vi "MainUI.vi"() -> ()   [LabVIEW 2016]
uses:
  Package Libraries/Message Queue/private/MessageQueue.MessageTypeDef.ctl
  Package ErrorHandling/ErrorHandling.lvclass/ErrorHandling.ctl
  Package ResourceControl/ViHandler/ViHandler.RunModes.ctl
  Package ErrorHandling/ErrorHandling.checkForErrorAndHandle.vi
  Package ErrorHandling/ErrorHandling.GetErrorHandler.vi
  <vilib>/Utility/error.llb/Clear Errors.vi
  Package Libraries/StringFunctions/StringFunctions_ReplaceAllBlindSigns.vi
  <vilib>/dlg_ctls.llb/Space Constant.vi
  Package Libraries/TimingFunctions/TimingFunctions_getUtcTimestamp.vi
  <vilib>/Utility/error.llb/Trim Whitespace.vi
  <vilib>/Utility/error.llb/Search and Replace Pattern.vi
  Package ErrorHandling/ErrorHandling.addLastErrorToFile.vi
  Package Simulation/Simulation Main/Simulation.Main.vi
  <vilib>/Utility/error.llb/Error Cluster From Error Code.vi
  Package ErrorHandling/ErrorHandling.lvclass
  <vilib>/ErrorRing/Error Ring.xnode
  Package ResourceControl/ViHandler/ViHandler.lvclass
  Package ResourceControl/ObjectHandler/ObjectHandler.lvclass
  Package Simulation/Simulation Main/Simulation.lvclass
panel:
  out "LastLoaded":string="LoadImportAssistant"
  out "NowLoaded":string="LoadImportAssistant"
  in  "PlaceHolder2Btn":bool
  in  "ParameterBtn":bool
  in  "ManualBtn":bool
  in  "DebugBtn":bool
  in  "ErrorHistoryBtn":bool
  in  "SimulationBtn":bool
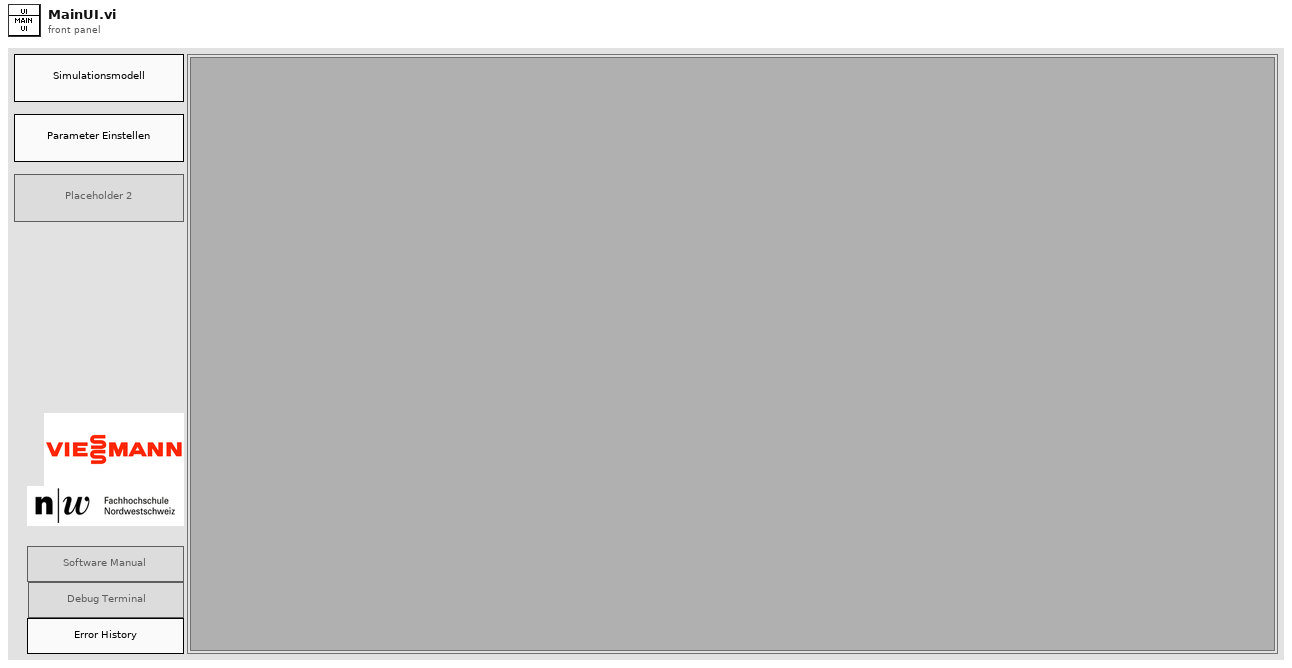
[diagram p1: front panel]
types:
  T1 = typedef "MessageQueue.MessageTypeDef.ctl" = cluster{"Message":string, "Data":variant}
  T2 = enum32{"Invalid", "Standard", "Closed", "Hidden", "Minimized", "Maximized"}
  T3 = enum8{"Enabled", "Disabled", "Disabled and Grayed Out"}
  T4 = typedef "ViHandler.lvclass/ViHandler.RunModes.ctl" = enum16{"FP Closed", "FP Open", "FP Open, Centered"}
  T5 = typedef "ViHandler.lvclass/ViHandler.ViInfo.ctl" = cluster{"ViName":string, "ViReference":refnum<vi>, "ViQueueName":string}
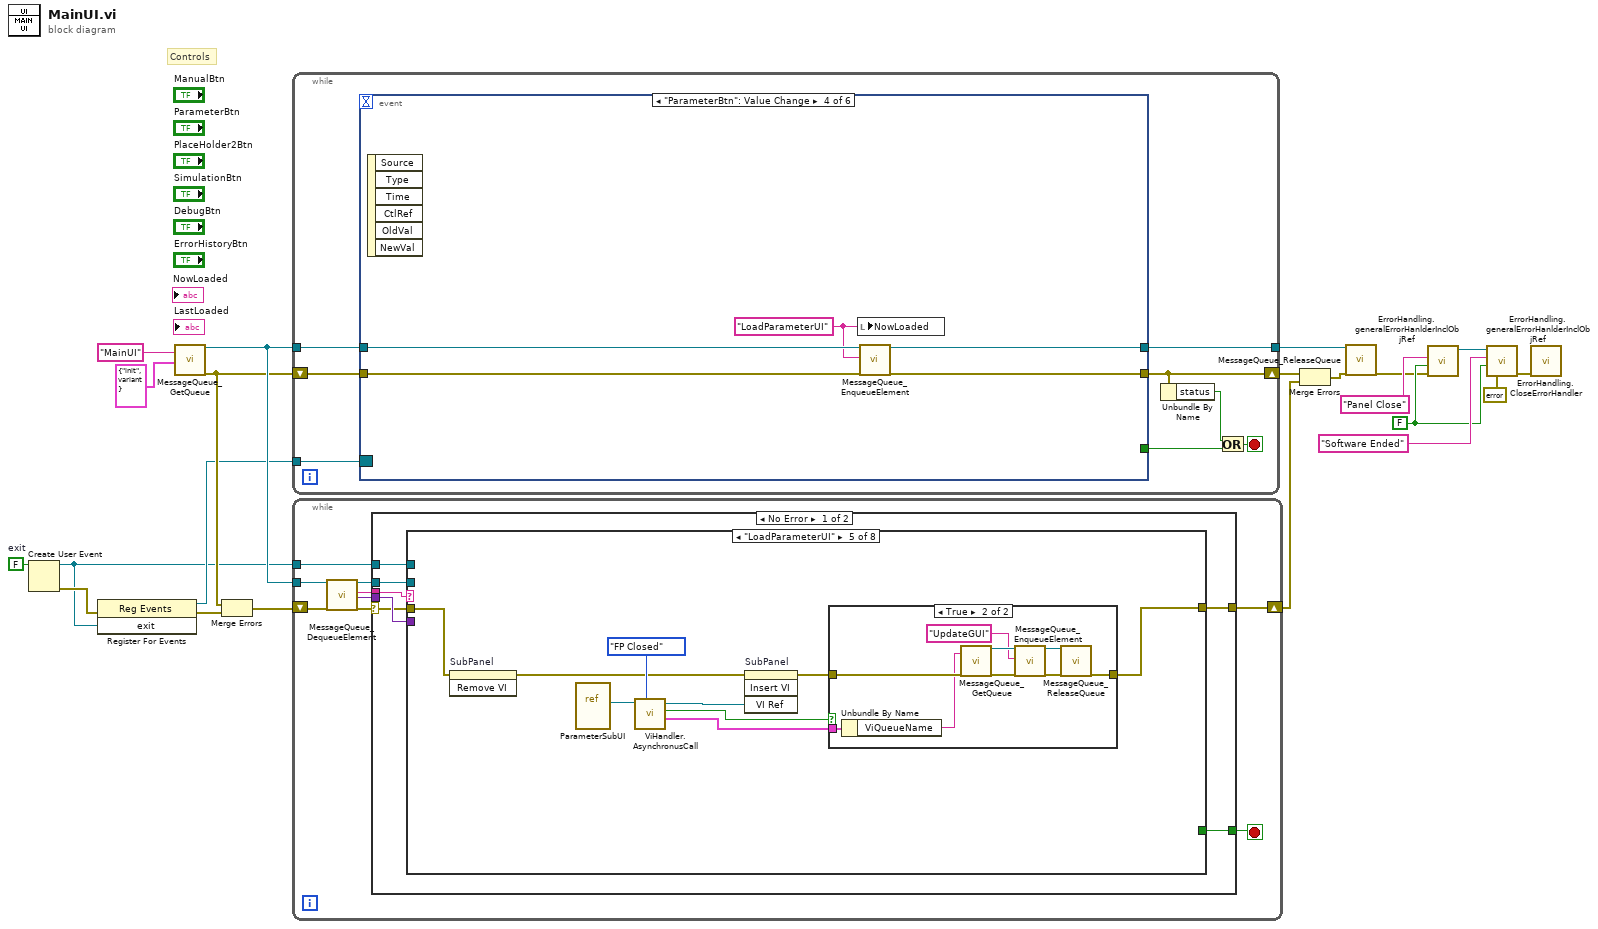
[diagram p0: block diagram]
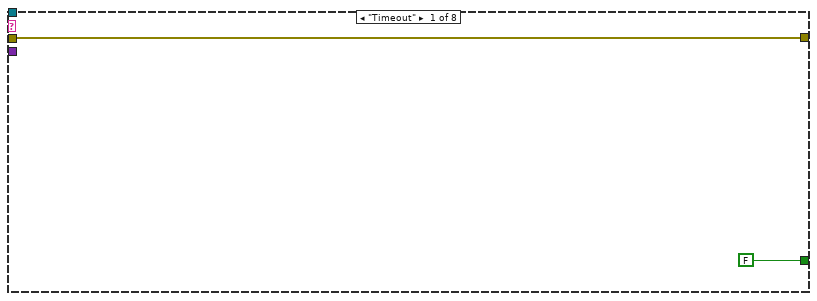
[diagram p2: hidden frame]
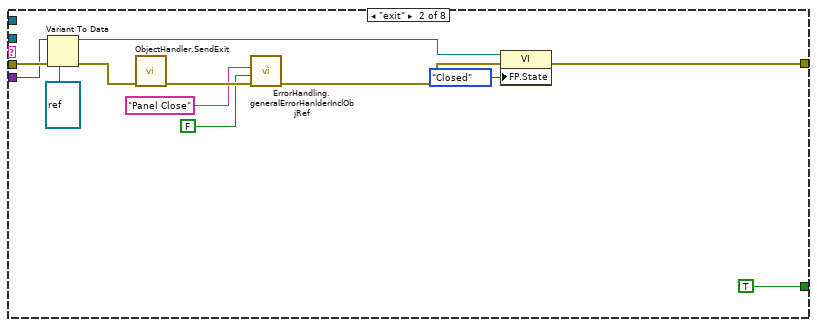
[diagram p3: hidden frame]
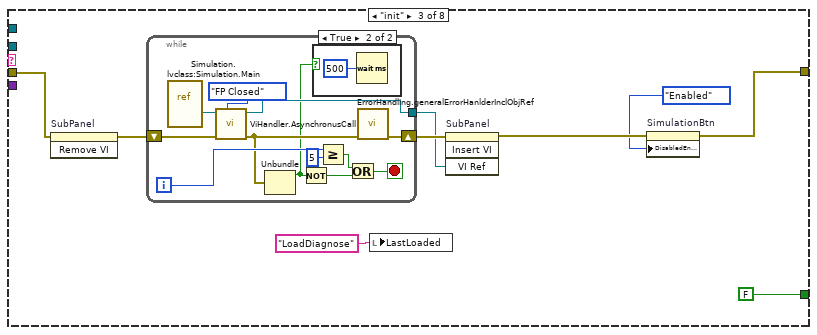
[diagram p4: hidden frame]
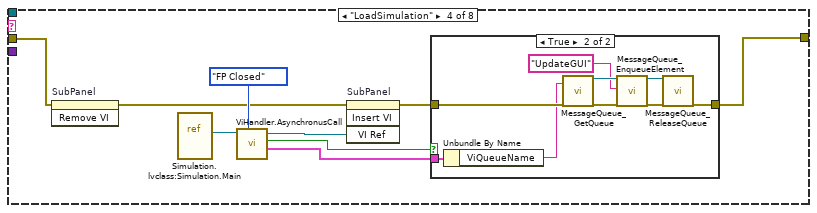
[diagram p6: hidden frame]
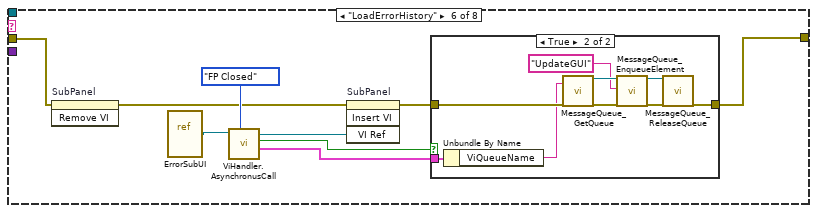
[diagram p9: hidden frame]
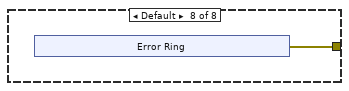
[diagram p12: hidden frame]
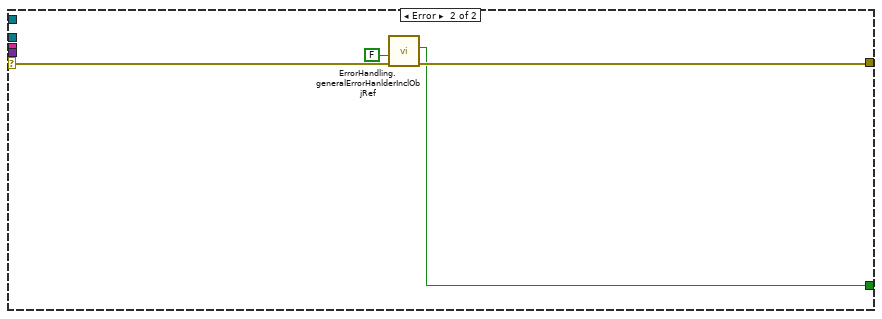
[diagram p13: hidden frame]
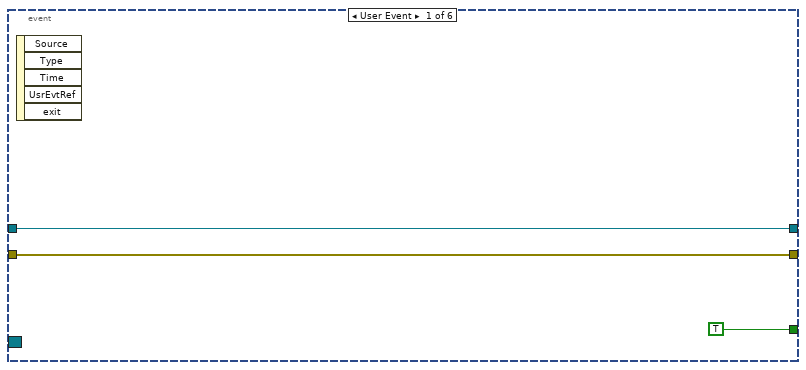
[diagram p14: hidden frame]
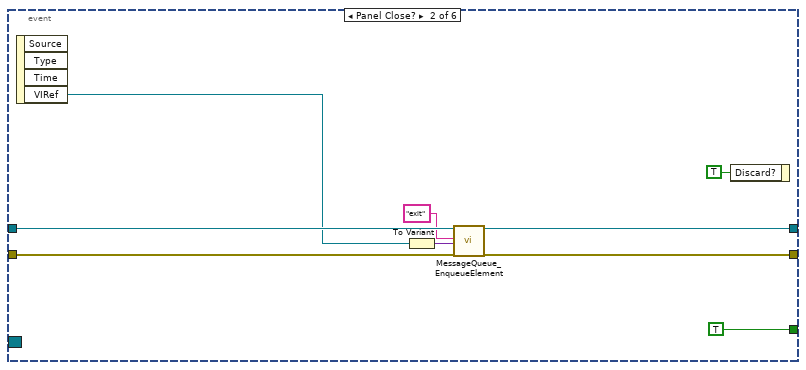
[diagram p15: hidden frame]
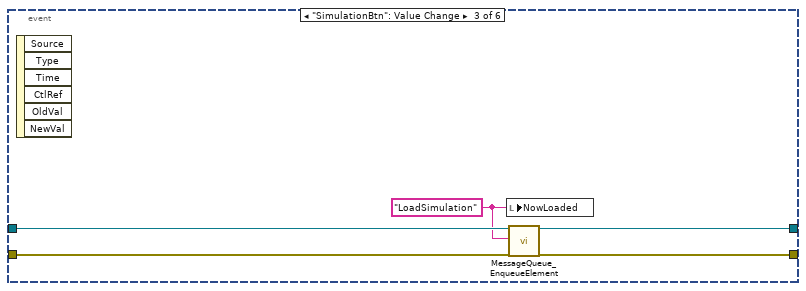
[diagram p16: hidden frame]
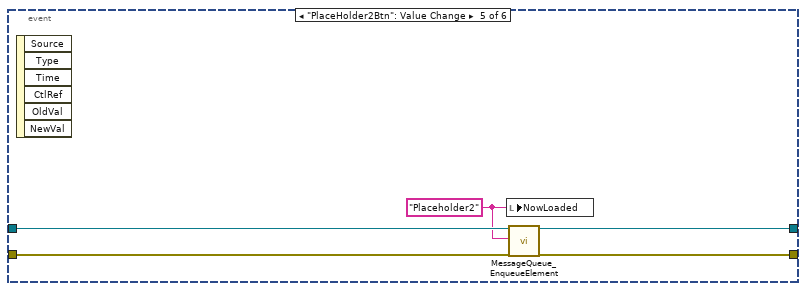
[diagram p17: hidden frame]
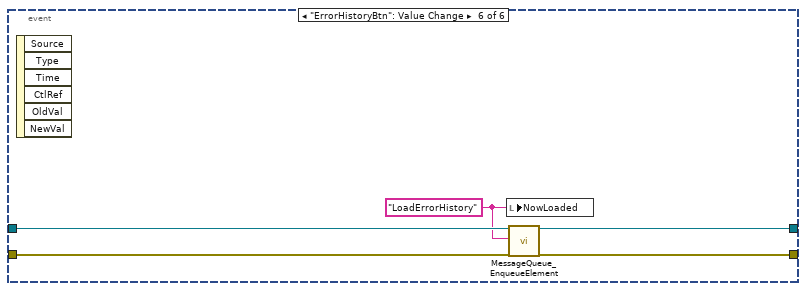
[diagram p18: hidden frame]
diagram:
  w3 = FALSE ("StopOnError")
  w14 = FALSE  # exit
  # "Controls"
  n1 = Create User Event(user event datatype=w14) -> (user event=w12:refnum<user-event>, error out=w13:errorcluster)  [unwired: 1 in]
  n2 = register-events(error in=w13, w12) -> (reference out=w16:refnum<event-registration>, error out=w18:errorcluster)  [unwired: 1 in]
  n3 = call "MessageQueue_GetQueue.vi"("Name"="MainUI", "OptionalInitValue"=T1 {"Message"="init", "Data"=variant}) -> ("QueueOut"=w20:refnum<queue>, "ErrorOut"=w17:errorcluster)  [unwired: 15 in, 1 out]
  n4 = Merge Errors(w17, w18) -> (w15:errorcluster)
  n5 = while {
    tunnel: w20 -> [w29]
    tunnel: [w28] -> w21
    shift-right: [w25] -> w9
    shift-left: w17 -> [w27]
    tunnel: w16 -> [w22]
    stop <- w24 stop-if-true
    n6 = event shown="[3] \"ParameterBtn\": Value Change" {
      selector: w22 -> [_ _ _ _ _ _]
      dyn-events: _ -> [_ _ _ _ _ _]
      timeout: _ -> [_ _ _ _ _ _]
      tunnel: w29 -> [w31 w41 w44 w49 w54 w59]
      tunnel: [w31 w40 w46 w51 w56 w61] -> w28
      tunnel: [w30 w33 w45 w50 w55 w60] -> w25
      tunnel: w27 -> [w30 w36 w43 w48 w53 w58]
      tunnel: [TRUE TRUE _ _ _ _] -> w26
      event User Event {
        n7 = event-data() -> ()  [unwired: 1 in, 5 out]
      }
      event Panel Close? {
        n8 = event-data() -> ("VIRef"=w34:refnum<vi>)  [unwired: 1 in, 3 out]
        n9 = To Variant(anything=w34) -> (Variant=w35:variant)
        n10 = call "MessageQueue_EnqueueElement.vi"("QueueIn"=w41, "Message"="exit", "Data"=w35, "ErrorIn"=w36) -> ("QueueOut"=w40:refnum<queue>, "ErrorOut"=w33:errorcluster)  [unwired: 14 in]
        n11 = event-data("Discard?"=TRUE) -> ()  [unwired: 1 in, 1 out]
      }
      event "SimulationBtn": Value Change {
        w42 = "LoadSimulation" ("Message")
        n12 = event-data() -> ()  [unwired: 1 in, 6 out]
        n13 = local write "NowLoaded"(w42) -> ()
        n14 = call "MessageQueue_EnqueueElement.vi"("QueueIn"=w44, "Message"=w42, "ErrorIn"=w43) -> ("QueueOut"=w46:refnum<queue>, "ErrorOut"=w45:errorcluster)  [unwired: 15 in]
      }
      event "ParameterBtn": Value Change {
        w47 = "LoadParameterUI" ("Message")
        n15 = event-data() -> ()  [unwired: 1 in, 6 out]
        n16 = local write "NowLoaded"(w47) -> ()
        n17 = call "MessageQueue_EnqueueElement.vi"("QueueIn"=w49, "Message"=w47, "ErrorIn"=w48) -> ("QueueOut"=w51:refnum<queue>, "ErrorOut"=w50:errorcluster)  [unwired: 15 in]
      }
      event "PlaceHolder2Btn": Value Change {
        w52 = "Placeholder2" ("Message")
        n18 = event-data() -> ()  [unwired: 1 in, 6 out]
        n19 = local write "NowLoaded"(w52) -> ()
        n20 = call "MessageQueue_EnqueueElement.vi"("QueueIn"=w54, "Message"=w52, "ErrorIn"=w53) -> ("QueueOut"=w56:refnum<queue>, "ErrorOut"=w55:errorcluster)  [unwired: 15 in]
      }
      event "ErrorHistoryBtn": Value Change {
        w57 = "LoadErrorHistory" ("Message")
        n21 = event-data() -> ()  [unwired: 1 in, 6 out]
        n22 = local write "NowLoaded"(w57) -> ()
        n23 = call "MessageQueue_EnqueueElement.vi"("QueueIn"=w59, "Message"=w57, "ErrorIn"=w58) -> ("QueueOut"=w61:refnum<queue>, "ErrorOut"=w60:errorcluster)  [unwired: 15 in]
      }
    }
    n24 = Unbundle By Name(w25) -> ("status"=w23:bool)
    n25 = Or(x=w23, y=w26) -> (x .or. y?=w24:bool)
  }
  n26 = while {
    tunnel: w20 -> [w70]
    tunnel: w12 -> [w63]
    shift-right: [w62] -> w10
    shift-left: w15 -> [w64]
    stop <- w65 stop-if-true
    n27 = call "MessageQueue_DequeueElement.vi"("QueueIn"=w70, "ErrorIn"=w64) -> ("QueueOut"=w68:refnum<queue>, "Message"=w67:string, "Data"=w66:variant, "ErrorOut"=w69:errorcluster)  [unwired: 13 in, 1 out]
    n28 = case shown="No Error" w69 {
      selector: w69 -> [w73 w181]
      tunnel: w68 -> [w77 _]
      tunnel: w67 -> [w76 _]
      tunnel: w66 -> [w75 _]
      tunnel: [w74 w179] -> w65
      tunnel: w63 -> [w72 _]
      tunnel: [w71 w180] -> w62
      frame No Error {
        n29 = case shown="\"LoadParameterUI\"" w76 {
          tunnel: w77 -> [_ _ _ _ _ _ _ _]
          tunnel: w75 -> [_ w83 _ _ _ _ _ _]
          tunnel: [FALSE TRUE FALSE _ _ _ _ _] -> w74
          tunnel: w73 -> [w78 w85 w94 w117 w136 w155 w171 _]
          tunnel: w72 -> [_ _ _ _ _ _ _ _]
          tunnel: [w78 w80 w93 w116 w135 w154 w171 w172] -> w71
          frame "Timeout" {
          }
          frame "exit" {
            n30 = Variant To Data(error in=w85, type=refnum<vi> refnum ("VIRef"), Variant=w83) -> (data=w81:refnum<vi>, error out=w84:errorcluster)
            n31 = call "ObjectHandler.SendExit.vi"("ErrorIn"=w84) -> ("ErrorOut"=w89:errorcluster)  [unwired: 10 in]
            n32 = call "ErrorHandling.generalErrorHanlderInclObjRef.vi"("error in"=w89, "StopOnError"=FALSE, "Comment(optional)"="Panel Close" ("Comment")) -> ("error out"=w88:errorcluster)  [unwired: 6 in, 2 out]
            n33 = property class="VI"(reference=w81, error in=w88, "FP.State"=T2."Closed" ("Front Panel Window:State")) -> (error out=w80:errorcluster)  [unwired: 1 out]
          }
          frame "init" {
            n34 = invoke on="SubPanel" class="SubPnl" method="Remove VI"(error in=w94) -> (error out=w96:errorcluster)  [unwired: 2 in, 2 out]
            n35 = while {
              tunnel: [w102] -> w95
              shift-right: [w103] -> w97
              shift-left: w96 -> [w110]
              i -> [w107]
              stop <- w105 stop-if-true
              n36 = vi-ref "Simulation.lvclass:Simulation.Main.vi"() -> (w112:refnum<vi>)
              n37 = call "ViHandler.AsynchronusCall.vi"("Modes"=ViHandler.RunModes."FP Closed", "Error In"=w110, "ViReference"=w112) -> ("error out"=w104:errorcluster, "ViReference"=w102:refnum<vi>)  [unwired: 5 in, 2 out]
              n38 = Unbundle(w104) -> ("status"=w101:bool)  [unwired: 2 out]
              n39 = Not(x=w101) -> (.not. x?=w109:bool)
              n40 = case shown="True" w101 {
                frame False {
                }
                frame True {
                  n41 = Wait (ms)(milliseconds to wait=u32 500) -> ()  [unwired: 1 out]
                }
              }
              n42 = Greater Or Equal?(x=w107, y=5) -> (x >= y?=w108:bool)
              n43 = Or(x=w108, y=w109) -> (x .or. y?=w105:bool)
              n44 = call "ErrorHandling.generalErrorHanlderInclObjRef.vi"("error in"=w104) -> ("error out"=w103:errorcluster)  [unwired: 8 in, 2 out]
            }
            n45 = local write "LastLoaded"("LoadDiagnose" ("Message")) -> ()
            n46 = invoke on="SubPanel" class="SubPnl" method="Insert VI"(error in=w97, "VI Ref"=w95) -> (error out=w99:errorcluster)  [unwired: 2 in, 3 out]
            n47 = property on="SimulationBtn" class="Bool"(error in=w99, "DisabledEnum"=T3."Enabled" ("Disabled")) -> (error out=w93:errorcluster)  [unwired: 1 in, 1 out]
          }
          frame "LoadSimulation" {
            n48 = invoke on="SubPanel" class="SubPnl" method="Remove VI"(error in=w117) -> (error out=w118:errorcluster)  [unwired: 2 in, 2 out]
            n49 = vi-ref "Simulation.lvclass:Simulation.Main.vi"() -> (w115:refnum<vi>)
            n50 = call "ViHandler.AsynchronusCall.vi"("Modes"=ViHandler.RunModes."FP Closed", "ViReference"=w115) -> ("ViInfo(OnlyIfFound=true)"=w122:T5, "ViFound?"=w121:bool, "ViReference"=w114:refnum<vi>)  [unwired: 6 in, 1 out]
            n51 = invoke on="SubPanel" class="SubPnl" method="Insert VI"(error in=w118, "VI Ref"=w114) -> (error out=w120:errorcluster)  [unwired: 2 in, 3 out]
            n52 = case shown="True" w121 {
              tunnel: w120 -> [w123 w132]
              tunnel: [w123 w129] -> w116
              tunnel: w122 -> [_ w128]
              frame False {
              }
              frame True {
                n53 = Unbundle By Name(w128) -> ("ViQueueName"=w125:string)
                n54 = call "MessageQueue_GetQueue.vi"("Name"=w125, "ErrorIn"=w132) -> ("QueueOut"=w127:refnum<queue>, "ErrorOut"=w131:errorcluster)  [unwired: 15 in, 1 out]
                n55 = call "MessageQueue_EnqueueElement.vi"("QueueIn"=w127, "Message"="UpdateGUI", "ErrorIn"=w131) -> ("QueueOut"=w126:refnum<queue>, "ErrorOut"=w130:errorcluster)  [unwired: 15 in]
                n56 = call "MessageQueue_ReleaseQueue.vi"("QueueIn"=w126, "ErrorIn"=w130) -> ("ErrorOut"=w129:errorcluster)  [unwired: 15 in, 2 out]
              }
            }
          }
          frame "LoadParameterUI" {
            n57 = invoke on="SubPanel" class="SubPnl" method="Remove VI"(error in=w136) -> (error out=w137:errorcluster)  [unwired: 2 in, 2 out]
            n58 = vi-ref "ParameterSubUI.vi"() -> (w134:refnum<vi>)
            n59 = call "ViHandler.AsynchronusCall.vi"("Modes"=ViHandler.RunModes."FP Closed", "ViReference"=w134) -> ("ViInfo(OnlyIfFound=true)"=w141:T5, "ViFound?"=w140:bool, "ViReference"=w133:refnum<vi>)  [unwired: 6 in, 1 out]
            n60 = invoke on="SubPanel" class="SubPnl" method="Insert VI"(error in=w137, "VI Ref"=w133) -> (error out=w139:errorcluster)  [unwired: 2 in, 3 out]
            n61 = case shown="True" w140 {
              tunnel: w139 -> [w142 w151]
              tunnel: [w142 w148] -> w135
              tunnel: w141 -> [_ w147]
              frame False {
              }
              frame True {
                n62 = Unbundle By Name(w147) -> ("ViQueueName"=w144:string)
                n63 = call "MessageQueue_GetQueue.vi"("Name"=w144, "ErrorIn"=w151) -> ("QueueOut"=w146:refnum<queue>, "ErrorOut"=w150:errorcluster)  [unwired: 15 in, 1 out]
                n64 = call "MessageQueue_EnqueueElement.vi"("QueueIn"=w146, "Message"="UpdateGUI", "ErrorIn"=w150) -> ("QueueOut"=w145:refnum<queue>, "ErrorOut"=w149:errorcluster)  [unwired: 15 in]
                n65 = call "MessageQueue_ReleaseQueue.vi"("QueueIn"=w145, "ErrorIn"=w149) -> ("ErrorOut"=w148:errorcluster)  [unwired: 15 in, 2 out]
              }
            }
          }
          frame "LoadErrorHistory" {
            n66 = invoke on="SubPanel" class="SubPnl" method="Remove VI"(error in=w155) -> (error out=w156:errorcluster)  [unwired: 2 in, 2 out]
            n67 = vi-ref "ErrorSubUI.vi"() -> (w153:refnum<vi>)
            n68 = call "ViHandler.AsynchronusCall.vi"("Modes"=ViHandler.RunModes."FP Closed", "ViReference"=w153) -> ("ViInfo(OnlyIfFound=true)"=w160:T5, "ViFound?"=w159:bool, "ViReference"=w152:refnum<vi>)  [unwired: 6 in, 1 out]
            n69 = invoke on="SubPanel" class="SubPnl" method="Insert VI"(error in=w156, "VI Ref"=w152) -> (error out=w158:errorcluster)  [unwired: 2 in, 3 out]
            n70 = case shown="True" w159 {
              tunnel: w158 -> [w161 w170]
              tunnel: [w161 w167] -> w154
              tunnel: w160 -> [_ w166]
              frame False {
              }
              frame True {
                n71 = Unbundle By Name(w166) -> ("ViQueueName"=w163:string)
                n72 = call "MessageQueue_GetQueue.vi"("Name"=w163, "ErrorIn"=w170) -> ("QueueOut"=w165:refnum<queue>, "ErrorOut"=w169:errorcluster)  [unwired: 15 in, 1 out]
                n73 = call "MessageQueue_EnqueueElement.vi"("QueueIn"=w165, "Message"="UpdateGUI", "ErrorIn"=w169) -> ("QueueOut"=w164:refnum<queue>, "ErrorOut"=w168:errorcluster)  [unwired: 15 in]
                n74 = call "MessageQueue_ReleaseQueue.vi"("QueueIn"=w164, "ErrorIn"=w168) -> ("ErrorOut"=w167:errorcluster)  [unwired: 15 in, 2 out]
              }
            }
          }
          frame "UpdateGUI" {
          }
          frame Default {
            n75 = xnode "Error Ring"() -> ("error out"=w172:errorcluster)
          }
        }
      }
      frame Error {
        n76 = call "ErrorHandling.generalErrorHanlderInclObjRef.vi"("error in"=w181, "StopOnError"=FALSE) -> ("error out"=w180:errorcluster, "Stop"=w179:bool)  [unwired: 7 in, 1 out]
      }
    }
  }
  n77 = Merge Errors(w9, w10) -> (w8:errorcluster)
  n78 = call "MessageQueue_ReleaseQueue.vi"("QueueIn"=w21, "ErrorIn"=w8) -> ("ErrorOut"=w1:errorcluster)  [unwired: 15 in, 2 out]
  n79 = call "ErrorHandling.generalErrorHanlderInclObjRef.vi"("error in"=w1, "StopOnError"=w3, "Comment(optional)"="Panel Close" ("Comment")) -> ("ErrorHandling out"=w5:refnum<data-value>)  [unwired: 6 in, 2 out]
  n80 = call "ErrorHandling.generalErrorHanlderInclObjRef.vi"("error in"=errorcluster {"status"=TRUE, "code"=0, "source"="Software Ended"}, "StopOnError"=w3, "Comment(optional)"="Software Ended" ("Comment"), "ErrorHandling(optional)"=w5) -> ("error out"=w7:errorcluster)  [unwired: 5 in, 2 out]
  n81 = call "ErrorHandling.CloseErrorHandler.vi"("ErrorIn"=w7) -> ()  [unwired: 10 in, 1 out]
